vi "tensao_e_voltagem.vi"(2 "T":dbl, 3 "th":dbl) -> (0 "Duty Cycle":dbl, 1 "Sentido":enum16{"Horário", "Anti-Horário"}(ring))   [LabVIEW 2018]
doc: "The myRIO Project template acquires acceleration data from the onboard accelerometer and displays the changes of acceleration values in a waveform chart."
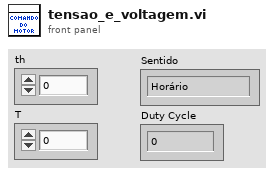
[diagram p1: front panel]
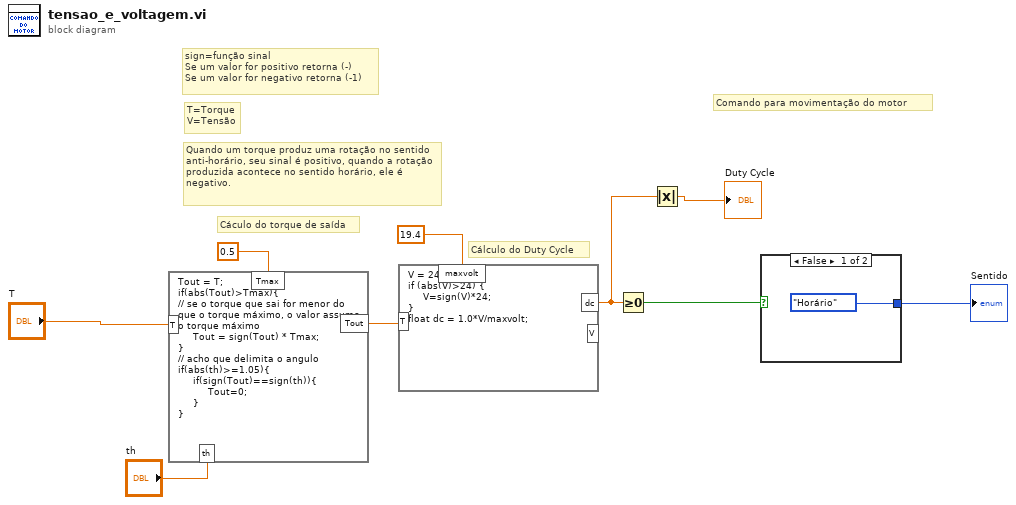
[diagram p0: block diagram]
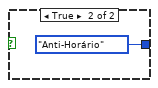
[diagram p2: hidden frame]
diagram:
  # "Quando um torque produz uma rotação no sentido anti-horário, seu sinal é positivo, quando a rotação produzida acontece no sentido horário, ele é negativo."
  # "sign=função sinal\nSe um valor for positivo retorna (-)\nSe um valor for negativo retorna (-1)"
  # "T=Torque\nV=Tensão"
  # "Comando para movimentação do motor"
  # "Cálculo do Duty Cycle"
  # "Cáculo do torque de saída"
  n1 = formula code="Tout = T;\nif(abs(Tout)>Tmax){ \n// se o torque que sai for menor do que o torque máximo, o valor assume o torque máximo\n     Tout = sign(Tout) * Tmax;\n}\n// acho que delimita o angulo\nif(abs(th)>=1.05){\n     if(sign(Tout)==sign(th)){\n          Tout=0;\n     }\n}"("Tmax"=0.5 ("input variable"), "T"="T", "th"="th") -> ("Tout"=w5:dbl)
  n2 = formula code="V = 24/3*T;\nif (abs(V)>24) {\n     V=sign(V)*24;\n}\nfloat dc = 1.0*V/maxvolt;"("maxvolt"=19.4 ("input variable"), "T"=w5) -> ("dc"=w4:dbl)  [unwired: 1 out]
  n3 = Greater Or Equal To 0?(x=w4) -> (x >= 0?=w7:bool)
  n4 = Absolute Value(x=w4) -> (abs(x)=→"Duty Cycle":dbl)
  n5 = case shown="False" w7 {
    tunnel: [enum16{"Horário", "Anti-Horário"}."Horário" enum16{"Horário", "Anti-Horário"}."Anti-Horário"] -> w2
    frame False {
    }
    frame True {
    }
  }
  "Sentido" <- w2
